vi "Create temporary file name.vi"(6 "Temporary Image File":T1=enum.".jpeg", 7 "Flush Files (F)":bool, 8 "error in (no error)":errorcluster, 9 "msec (F)":bool, 10 "hh:mm:ss (false)":bool, 11 "Dir path":path) -> (0 "error out":errorcluster, 3 "File path":path)   [LabVIEW 2012]
doc: "Version 1.0\nDeveloped by Jean-Marc Simard\nCopyright © 2010, Exaprom Inc.\nAll rights reserved.\nLicense: BSD"
uses:
  Controls/Temporary Image File.ctl
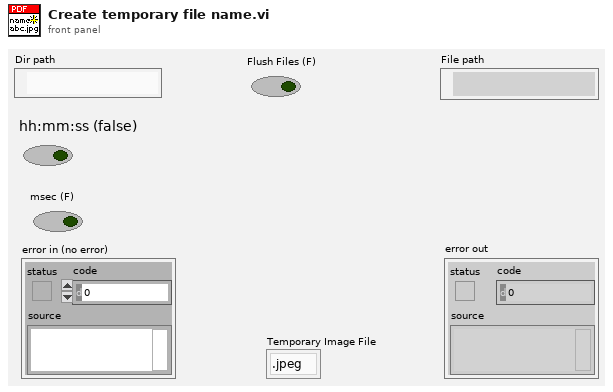
[diagram p1: front panel]
types:
  T1 = typedef "Temporary Image File.ctl" = enum16{".bmp", ".jpeg", ".png", ".pdf", "No File"}
  T2 = typedef "LVDateTimeRec.ctl" = cluster{"fractional second":dbl, "second":i32, "minute":i32, "hour":i32, "day of month":i32, "month":i32, "year":i32, "day of week":i32, "day of year":i32, "DST":i32}
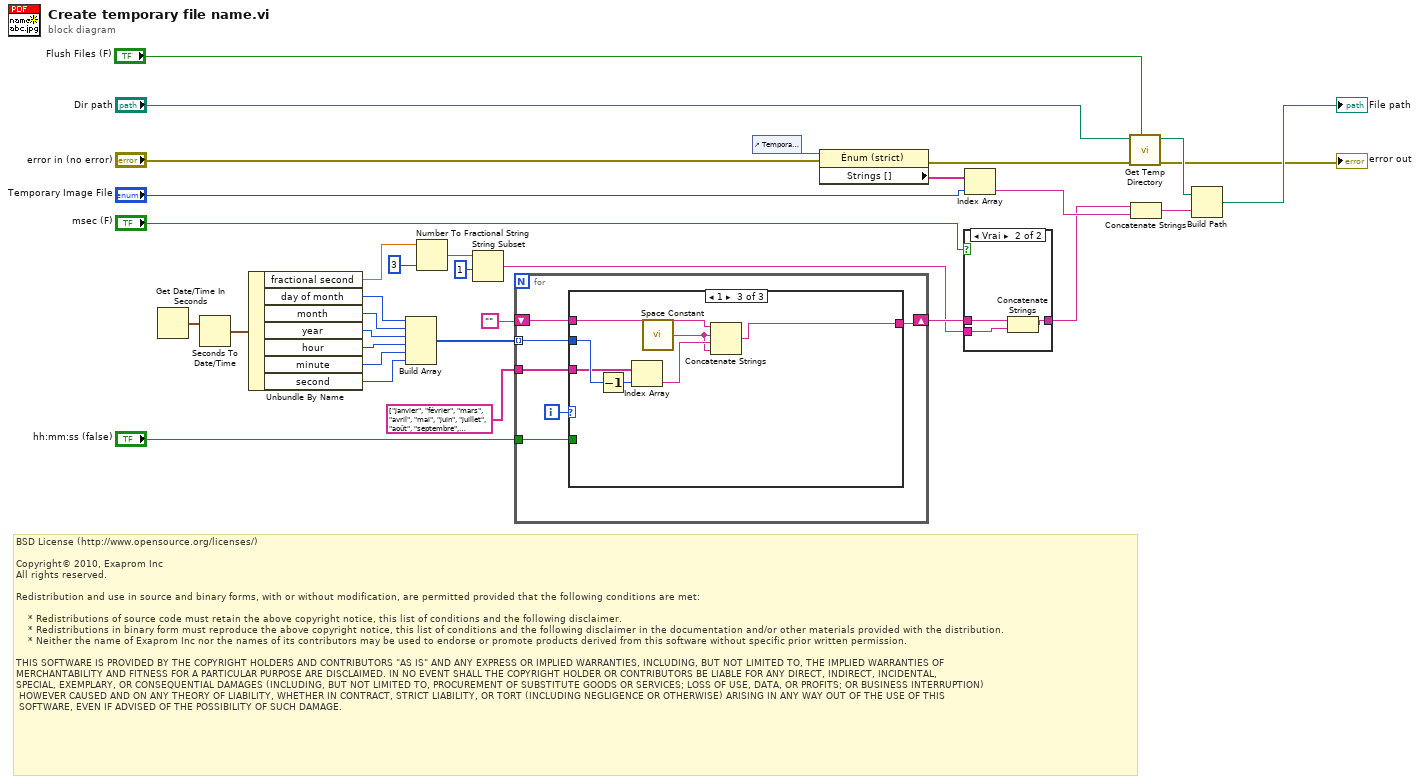
[diagram p0: block diagram]
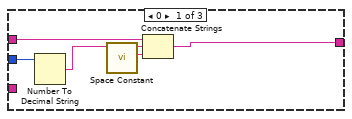
[diagram p3: hidden frame]
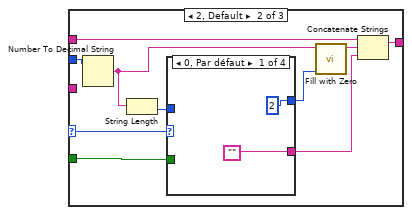
[diagram p4: hidden frame]
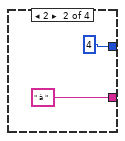
[diagram p5: hidden frame]
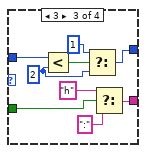
[diagram p6: hidden frame]
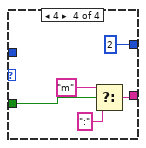
[diagram p7: hidden frame]
diagram:
  # "BSD License (http://www.opensource.org/licenses/)\n\nCopyright© 2010, Exaprom Inc\nAll rights reserved.\n\nRedistribution and use in source and binary forms, with or without modification, are permitted provided that the following conditions are met:\n\n    * Redistributions of source code must retain the above copyright notice, this list of conditions and the following disclaimer.\n    * Redistributions in binary form must reproduce the above copyright notice, this list of conditions and the following disclaimer in the documentation and/or other materials provided with the distribution.\n    * Neither the name of Exaprom Inc nor the names of its contributors may be used to endorse or promote products derived from this software without specific prior written permission.\n\nTHIS SOFTWARE IS PROVIDED BY THE COPYRIGHT HOLDERS AND CONTRIBUTORS \"AS IS\" AND ANY EXPRESS OR IMPLIED WARRANTIES, INCLUDING, BUT NOT LIMITED TO, THE IMPLIED WARRANTIES OF \nMERCHANTABILITY AND FITNESS FOR A PARTICULAR PURPOSE ARE DISCLAIMED. IN NO EVENT SHALL THE COPYRIGHT HOLDER OR CONTRIBUTORS BE LIABLE FOR ANY DIRECT, INDIRECT, INCIDENTAL,\nSPECIAL, EXEMPLARY, OR CONSEQUENTIAL DAMAGES (INCLUDING, BUT NOT LIMITED TO, PROCUREMENT OF SUBSTITUTE GOODS OR SERVICES; LOSS OF USE, DATA, OR PROFITS; OR BUSINESS INTERRUPTION)\n HOWEVER CAUSED AND ON ANY THEORY OF LIABILITY, WHETHER IN CONTRACT, STRICT LIABILITY, OR TORT (INCLUDING NEGLIGENCE OR OTHERWISE) ARISING IN ANY WAY OUT OF THE USE OF THIS\n SOFTWARE, EVEN IF ADVISED OF THE POSSIBILITY OF SUCH DAMAGE."
  n1 = Get Date/Time In Seconds() -> (seconds since 1Jan1904=w32:timestamp)
  n2 = Seconds To Date/Time(time stamp (now)=w32) -> (date time rec=w31:T2)  [unwired: 1 out]
  n3 = Unbundle By Name(w31) -> ("fractional second"=w20:dbl, "day of month"=w30:i32, "month"=w29:i32, "year"=w28:i32, "hour"=w27:i32, "minute"=w26:i32, "second"=w25:i32)
  n4 = Build Array(w30, w29, w28, w27, w26, w25) -> (w24:i32[])
  n5 = Number To Fractional String(number=w20, precision (6)=i16 3) -> (F-format string=w19:string)  [unwired: 2 out]
  n6 = String Subset(string=w19, offset (0)=1) -> (substring=w15:string)  [unwired: 1 out]
  n7 = for {
    tunnel: w24 -> [w35] mode=indexing
    tunnel: string[] ["janvier", "février", "mars", "avril", "mai", "juin", "juillet", "août", "septembre", "octobre", "novembre", "décembre"] -> [w37]
    shift-right: [w34] -> w21
    shift-left: "" -> [w36]
    tunnel: "hh:mm:ss (false)" -> [w33]
    i -> [w38]
    n8 = case shown="1" w38 {
      selector: w38 -> [_ w50 _]
      tunnel: w37 -> [_ _ w77]
      tunnel: w36 -> [w42 w52 w76]
      tunnel: w35 -> [w43 w53 w78]
      tunnel: [w41 w51 w74] -> w34
      tunnel: w33 -> [_ w48 _]
      frame 0 {
        n9 = Number To Decimal String(number=w43) -> (decimal integer string=w40:string)  [unwired: 1 out]
        n10 = call <vilib>:"Space Constant.vi"() -> ("String"=w39:string)
        n11 = Concatenate Strings(w42, w40, w39) -> (w41:string)
      }
      frame 2, Default {
        n12 = Number To Decimal String(number=w53) -> (decimal integer string=w45:string)  [unwired: 1 out]
        n13 = String Length(string=w45) -> (length=w44:i32)
        n14 = case shown="0, Par défaut" w50 {
          tunnel: ["" " à " w64 w69] -> w49
          tunnel: w48 -> [_ _ w65 w68]
          tunnel: [2 4 w60 2] -> w46
          tunnel: w44 -> [_ _ w62 _]
          frame 0, Default {
          }
          frame 2 {
          }
          frame 3 {
            w59 = 2 ("y")
            n15 = Less?(x=w62, y=w59) -> (x < y?=w61:bool)
            n16 = Select(t=1, s=w61, f=w59) -> (s? t:f=w60:i32)
            n17 = Select(t="h", s=w65, f=":") -> (s? t:f=w64:string)
          }
          frame 4 {
            n18 = Select(t="m", s=w68, f=":") -> (s? t:f=w69:string)
          }
        }
        n19 = call "Fill with Zero.vi"("Nbre caractères"=w46, "String IN"=w45) -> ("String OUT"=w47:string)  [unwired: 9 out]
        n20 = Concatenate Strings(w52, w47, w49) -> (w51:string)
      }
      frame 1 {
        n21 = Decrement(x=w78) -> (x-1=w73:i32)
        n22 = Index Array(array=w77, index=w73) -> (element=w75:string)
        n23 = call <vilib>:"Space Constant.vi"() -> ("String"=w72:string)
        n24 = Concatenate Strings(w76, w72, w75, w72) -> (w74:string)
      }
    }
  }
  n25 = control-ref of="Temporary Image File"() -> (w11:refnum<vi>)
  n26 = property class="Énum (strict)"(reference=w11, error in="error in (no error)") -> (error out=w7:errorcluster, "Strings []"=w10:string[])  [unwired: 1 out]
  n27 = case shown="Vrai" "msec (F)" {
    tunnel: w21 -> [w79 w82]
    tunnel: [w79 w81] -> w8
    tunnel: w15 -> [_ w80]
    frame False {
    }
    frame True {
      n28 = Concatenate Strings(w82, w80) -> (w81:string)
    }
  }
  n29 = Index Array(array=w10, index="Temporary Image File") -> (element=w9:string)
  n30 = call "Get Temp Directory.vi"("Flush Files (F)"="Flush Files (F)", "error in (no error)"=w7, "Dir path"="Dir path") -> ("error out"=→"error out":errorcluster, "created path"=w12:path)  [unwired: 7 out]
  n31 = Concatenate Strings(w8, w9) -> (w13:string)
  n32 = Build Path(base path=w12, name or relative path=w13) -> (appended path=→"File path":path)
